vi "Detect USB Drives (subVI).vi"(8 "error in (no error)":errorcluster) -> (0 "error out":errorcluster, 3 "USB drive's list":path[](array[path]))   [LabVIEW 2018]
uses:
  C:/Windows/System32/kernel32.dll
panel:
  out "Enum":T1(ring)
  out "Flash Drive Path":path
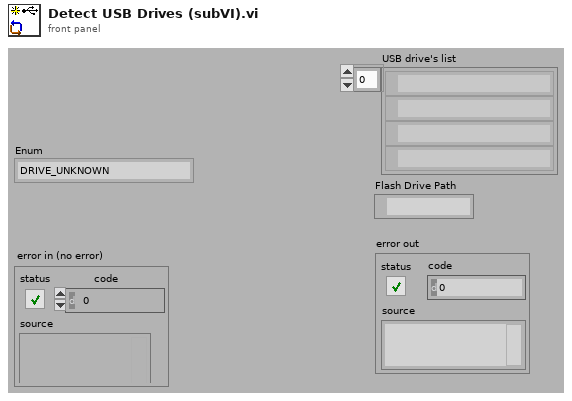
[diagram p1: front panel]
types:
  T1 = enum8{"DRIVE_UNKNOWN", "DRIVE_NO_ROOT_DIR", "DRIVE_REMOVABLE", "DRIVE_FIXED", "DRIVE_REMOTE", "DRIVE_CDROM", "DRIVE_RAMDISK"}
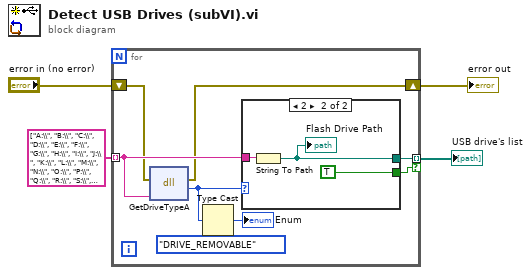
[diagram p0: block diagram]
diagram:
  n1 = for {
    tunnel: string[] ["A:\\", "B:\\", "C:\\", "D:\\", "E:\\", "F:\\", "G:\\", "H:\\", "I:\\", "J:\\", "K:\\", "L:\\", "M:\\", "N:\\", "O:\\", "P:\\", "Q:\\", "R:\\", "S:\\", "T:\\", "U:\\", "V:\\", "W:\\", "X:\\", "Y:\\", "Z:\\"] ("array of strings") -> [w12] mode=indexing
    tunnel: [w9] -> w3 mode=indexing if=w8
    shift-right: [w5] -> w1
    shift-left: "error in (no error)" -> [w6]
    n2 = dll-call lib="C:/Windows/System32/kernel32.dll" fn="GetDriveTypeA"(error in=w6, "arg1"=w12) -> (error out=w5:errorcluster, "return type"=w7:u32)  [unwired: 3 in, 1 out]
    n3 = Type Cast(type=T1."DRIVE_REMOVABLE" ("Enum"), x=w7) -> (*(type *) &x=→"Enum":T1)
    n4 = case shown="2" w7 {
      tunnel: w12 -> [_ w15]
      tunnel: [_ TRUE] -> w8
      tunnel: [_ w13] -> w9
      frame Default {
      }
      frame 2 {
        n5 = String To Path(string=w15) -> (path=w13:path)
        "Flash Drive Path" <- w13
      }
    }
  }
  "USB drive's list" <- w3
  "error out" <- w1
